vi "Dashboard Main.vi"() -> ()   [LabVIEW 2011]
panel:
  out "Shoot Now!":bool
  out "Shooter Angle":dbl
  out "Potentiometer":cluster{"Pot Raw":dbl, "Pot Angle":dbl}
  out "Locked On":bool
  out "Indexer":T1
  out "Shooter RPM":dbl
  out "Loaded":bool
  in  "Viewer 2":enum32{"Camera Image 2"}(tab)
  in  "Video Enable 2":bool=TRUE
  out "Camera Image 3":T2(plugin-control)
  out "Image Error Message 2":string="Timeout in Camera Communications"
  out "Bridge Balanced":bool
  out "CountDown":dbl format="%#_5g"
  out "Camera":T3
  in  "Viewer":enum32{"Camera Image"}(tab)
  in  "Video Enable":bool=TRUE
  out "Camera Image":T2(plugin-control)
  out "Dashboard Datatype Warning":string="Warning: The Dashboard Datatype used by the robot project and this dashboard do not match.\nSee diagram for more details."
  out "Robot IP Address":string
  out "Image Error Message":string="Timeout in Camera Communications"
  # "Communications"
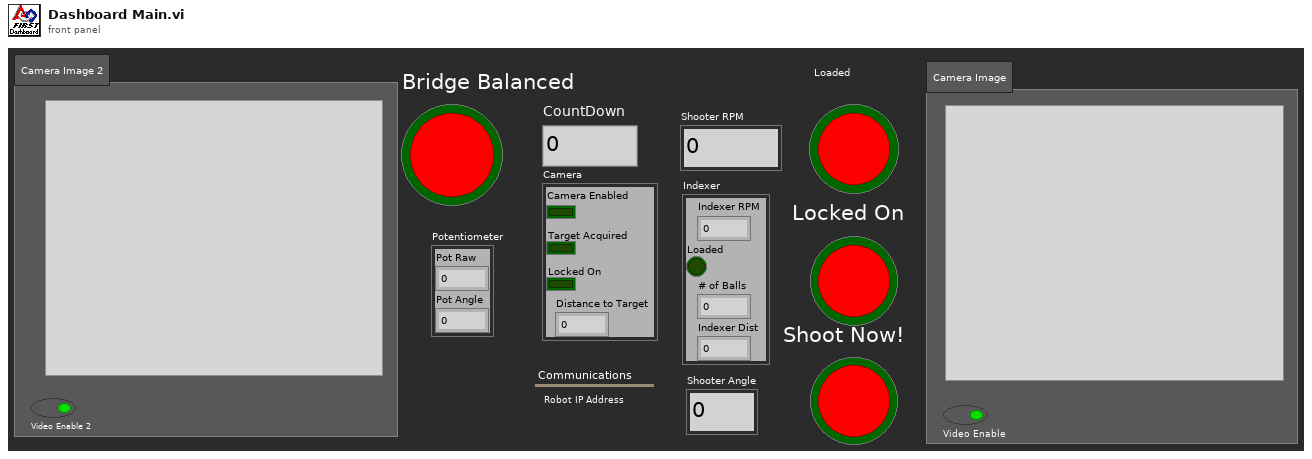
[diagram p1: front panel]
types:
  T1 = cluster{"Indexer RPM":dbl, "Loaded":bool, "# of Balls":dbl, "Indexer Dist":dbl}
  T2 = typedef "IMAQ Image.ctl" = refnum<image>
  T3 = cluster{"Locked On":bool, "Target Acquired":bool, "Camera Enabled":bool, "Distance to Target":dbl}
  T4 = cluster{"Robot Outputs":cluster{"Shooter":cluster{"Shooter RPM":dbl, "Shooter Angle":dbl, "Shooter Power":dbl, "Shooter Enabled":bool}, "Indexer":cluster{"Indexer RPM":dbl, "Loaded":bool, "# of Balls":dbl, "Indexer Dist":dbl}, "Camera":cluster{"Locked On":bool, "Target Acquired":bool, "Camera Enabled":bool, "Distance to Target":dbl}, "Potentiometer":cluster{"Pot Raw":dbl, "Pot Angle":dbl}, "Others":cluster{"CountDown":dbl, "Bridge Balance":bool, "PID Stable":bool}}}
  T5 = typedef "Image Type" = u32
  T6 = typedef "LVRectTypeDef.ctl" = cluster{"left":i16, "top":i16, "right":i16, "bottom":i16}
  T7 = cluster{"Competition mode":bool, "Robot Link":bool, "Autonomous":bool, "Enabled":bool, "E-Stop":bool}
  T8 = cluster{"Shooter":cluster{"Shooter RPM":dbl, "Shooter Angle":dbl, "Shooter Power":dbl, "Shooter Enabled":bool}, "Indexer":cluster{"Indexer RPM":dbl, "Loaded":bool, "# of Balls":dbl, "Indexer Dist":dbl}, "Camera":cluster{"Locked On":bool, "Target Acquired":bool, "Camera Enabled":bool, "Distance to Target":dbl}, "Potentiometer":cluster{"Pot Raw":dbl, "Pot Angle":dbl}, "Others":cluster{"CountDown":dbl, "Bridge Balance":bool, "PID Stable":bool}}
  T9 = cluster{"Shooter RPM":dbl, "Shooter Angle":dbl, "Shooter Power":dbl, "Shooter Enabled":bool}
  T10 = cluster{"CountDown":dbl, "Bridge Balance":bool, "PID Stable":bool}
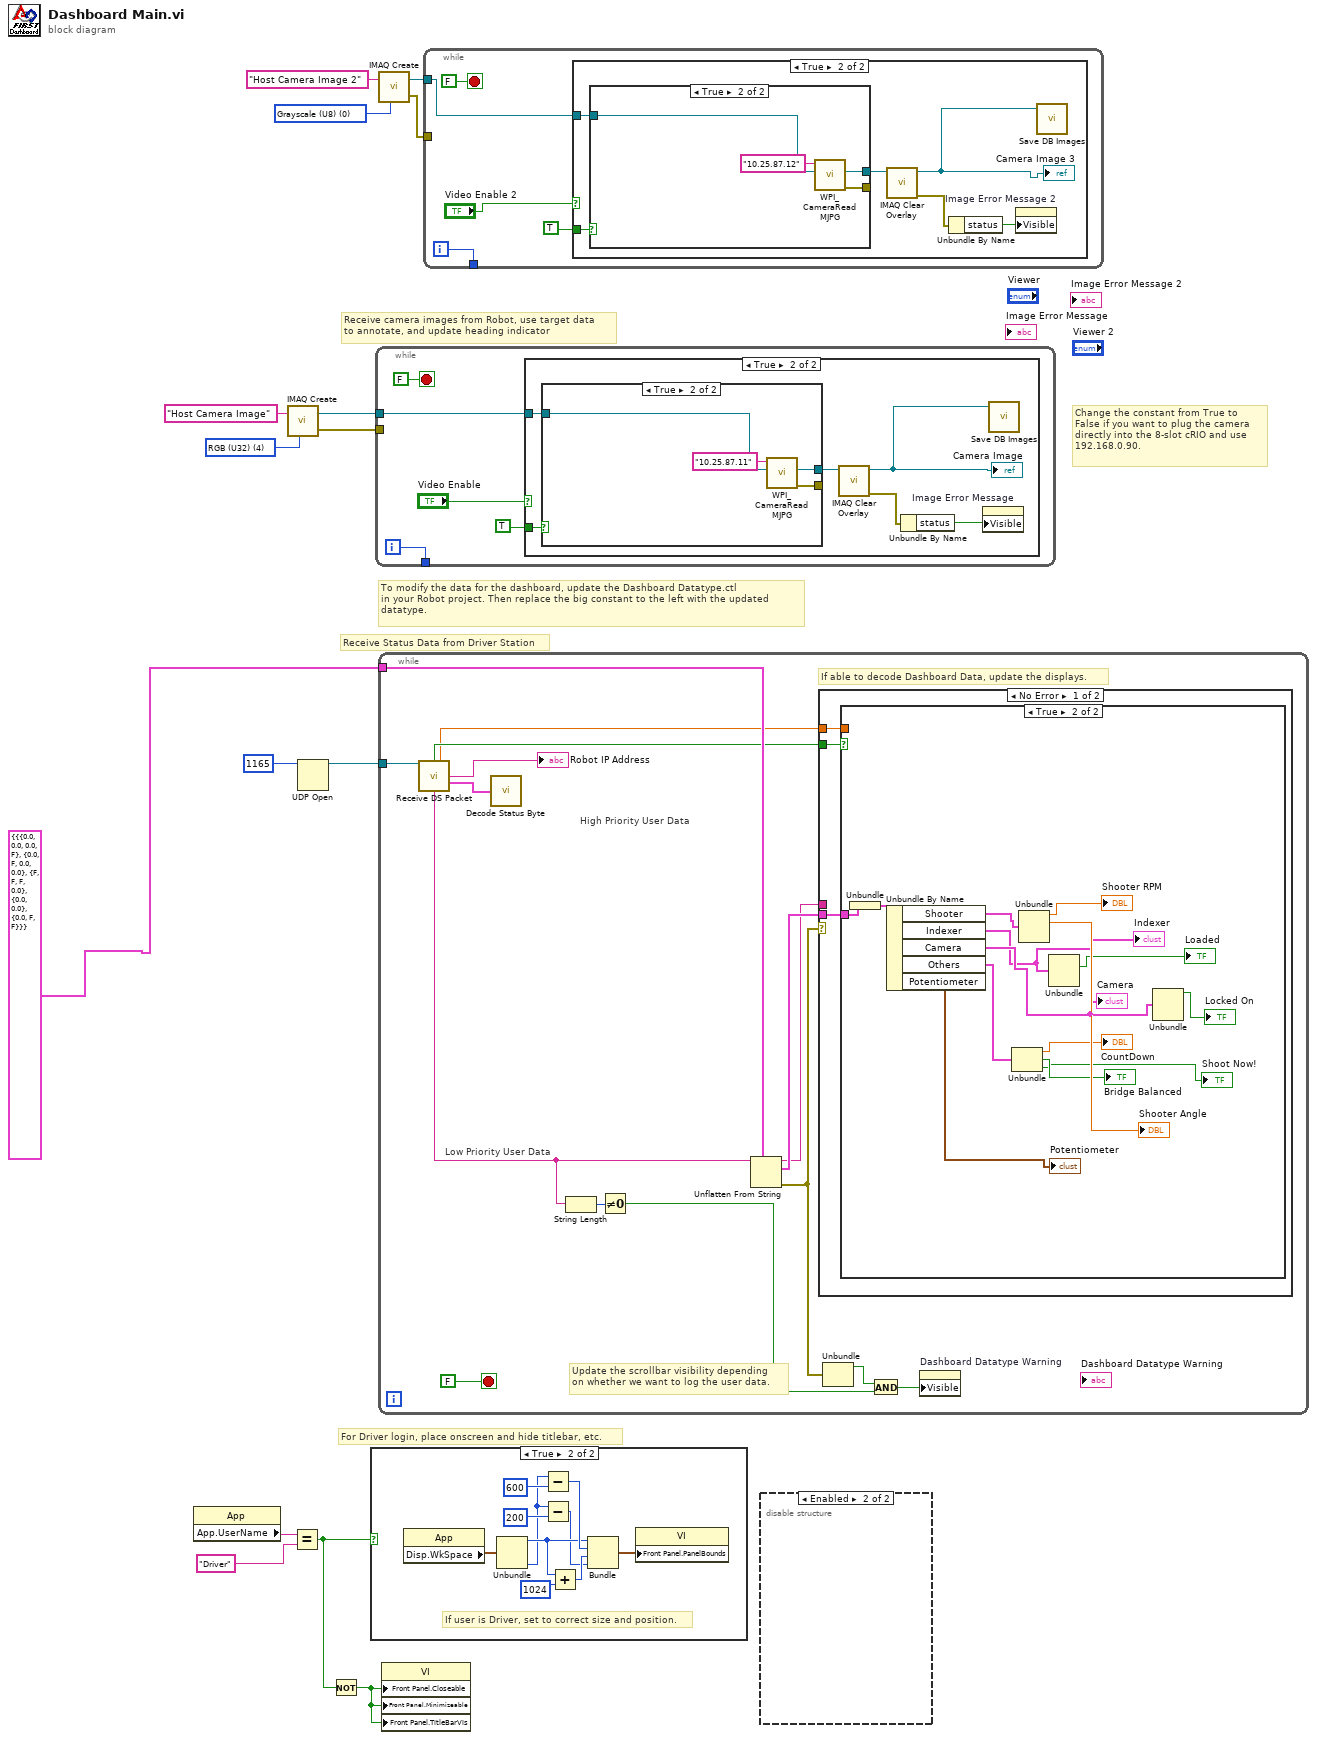
[diagram p0: block diagram]
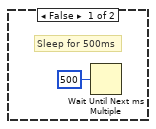
[diagram p2: hidden frame]
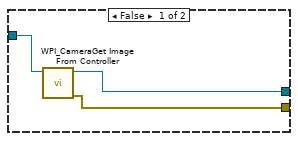
[diagram p3: hidden frame]
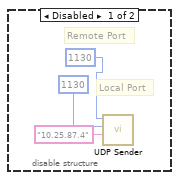
[diagram p4: hidden frame]
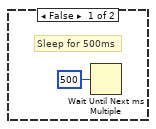
[diagram p8: hidden frame]
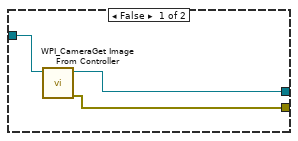
[diagram p9: hidden frame]
diagram:
  w5 = T5 0 items=["Grayscale (U8)", "Grayscale (I16)", "Grayscale (SGL)", "Complex (CSG)", "RGB (U32)", "HSL (U32)", "RGB (U64)"] ("Image Type")
  w13 = T5 4 items=["Grayscale (U8)", "Grayscale (I16)", "Grayscale (SGL)", "Complex (CSG)", "RGB (U32)", "HSL (U32)", "RGB (U64)"] ("Image Type")
  # "Change the constant from True to\nFalse if you want to plug the camera\ndirectly into the 8-slot cRIO and use\n192.168.0.90."
  # "For Driver login, place onscreen and hide titlebar, etc."
  # "To modify the data for the dashboard, update the Dashboard Datatype.ctl\nin your Robot project. Then replace the big constant to the left with the updated\ndatatype."
  # "Receive Status Data from Driver Station"
  # "Receive camera images from Robot, use target data\nto annotate, and update heading indicator"
  n1 = property class="App"() -> ("App.UserName"=w8:string)  [unwired: 2 in, 2 out]
  n2 = call "IMAQ Create"("Image Name"="Host Camera Image", "Image Type"=w13) -> ("New Image"=w11:T2, "error out"=w10:errorcluster)  [unwired: 2 in, 1 out]
  n3 = Equal?(x=w8, y="Driver") -> (x = y?=w7:bool)
  n4 = UDP Open(11:u16 1165 ("port")) -> (port=w14:refnum<k16>)  [unwired: 2 in, 4 out]
  n5 = Not(x=w7) -> (.not. x?=w6:bool)
  n6 = case shown="True" w7 {
    frame False {
    }
    frame True {
      # "If user is Driver, set to correct size and position."
      n7 = property class="App"() -> ("Disp.WkSpace"=w25:T6)  [unwired: 2 in, 2 out]
      n8 = Unbundle(w25) -> ("left"=w20:i16, "bottom"=w16:i16)  [unwired: 2 out]
      n9 = Subtract(x=w16, y=600) -> (x-y=w22:i32)
      n10 = Subtract(x=w16, y=200) -> (x-y=w17:i32)
      n11 = Add(x=w20, y=1024) -> (x+y=w21:i32)
      n12 = Bundle("left"=w20, w22, w21, w17) -> (w24:cluster{"left":i16, i32, i32, i32})  [unwired: 1 out]
      n13 = property class="VI"("Front Panel.PanelBounds"=w24) -> ()  [unwired: 2 in, 2 out]
    }
  }
  n14 = while {
    tunnel: w11 -> [w29]
    tunnel: w10 -> [_]
    tunnel: [w26] -> _
    i -> [w26]
    stop <- FALSE stop-if-true
    n15 = case shown="True" "Video Enable" {
      tunnel: w29 -> [_ w37]
      tunnel: TRUE -> [_ w34]
      frame False {
        # "Sleep for 500ms"
        n16 = Wait Until Next ms Multiple(millisecond multiple=u32 500) -> ()  [unwired: 1 out]
      }
      frame True {
        n17 = case shown="True" w34 {
          tunnel: w37 -> [w40 w44]
          tunnel: [w38 w42] -> _
          tunnel: [w39 w43] -> w35
          frame False {
            n18 = call <vilib>:"WPI_CameraGet Image From Controller.vi"("Image"=w40) -> ("error out"=w38:errorcluster, "Image Out"=w39:T2)  [unwired: 3 in, 6 out]
          }
          frame True {
            n19 = call <vilib>:"WPI_CameraRead MJPG.vi"("Image"=w44, "address"="10.25.87.11") -> ("error out"=w42:errorcluster, "Image Out"=w43:T2)  [unwired: 8 in]
          }
        }
        n20 = call "IMAQ Clear Overlay"("Image"=w35) -> ("error out"=w36:errorcluster, "Image Out"=w32:T2)  [unwired: 2 in, 7 out]
        "Camera Image" <- w32
        n21 = Unbundle By Name(w36) -> ("status"=w33:bool)
        n22 = property on="Image Error Message" class="Str"("Visible"=w33) -> ()  [unwired: 2 in, 2 out]
        n23 = call "Save DB Images.vi"("Image"=w32) -> ()  [unwired: 2 in, 1 out]
      }
    }
  }
  n24 = call "IMAQ Create"("Image Name"="Host Camera Image 2", "Image Type"=w5) -> ("New Image"=w3:T2, "error out"=w2:errorcluster)  [unwired: 2 in, 1 out]
  n25 = while {
    tunnel: w14 -> [w57]
    tunnel: T4 {"Robot Outputs"={"Shooter"={"Shooter RPM"=0.0, "Shooter Angle"=0.0, "Shooter Power"=0.0, "Shooter Enabled"=FALSE}, "Indexer"={"Indexer RPM"=0.0, "Loaded"=FALSE, "# of Balls"=0.0, "Indexer Dist"=0.0}, "Camera"={"Locked On"=FALSE, "Target Acquired"=FALSE, "Camera Enabled"=FALSE, "Distance to Target"=0.0}, "Potentiometer"={"Pot Raw"=0.0, "Pot Angle"=0.0}, "Others"={"CountDown"=0.0, "Bridge Balance"=FALSE, "PID Stable"=FALSE}}} ("Dashboard Data") -> [w56]
    stop <- FALSE stop-if-true
    # "High Priority User Data"
    # "Low Priority User Data"
    # "Update the scrollbar visibility depending\non whether we want to log the user data."
    # "If able to decode Dashboard Data, update the displays."
    n26 = call "Receive DS Packet.vi"("Recv Socket"=w57) -> ("New Dashboard Data"=w53:bool, "Battery"=w45:sgl, "Robot IP Address"=→"Robot IP Address":string, "Status"=w58:T7, "Low Priority User Data"=w46:string)  [unwired: 1 in, 9 out]
    n27 = call "Decode Status Byte.vi"("Status Byte"=w58) -> ()  [unwired: 2 out]
    n28 = String Length(string=w46) -> (length=w48:i32)
    n29 = Not Equal To 0?(x=w48) -> (x != 0?=w51:bool)
    n30 = Unflatten From String(type=w56, binary string=w46) -> (rest of the binary string=w49:string, value=w55:T4, error out=w54:errorcluster)  [unwired: 1 in, 2 out]
    n31 = case shown="No Error" w54 {
      tunnel: w55 -> [w62 _]
      tunnel: w53 -> [w61 _]
      tunnel: w49 -> [_ _]
      tunnel: w45 -> [w60 _]
      frame No Error {
        n32 = case shown="True" w61 {
          tunnel: w62 -> [_ w76]
          tunnel: w60 -> [_ _]
          frame False {
            # "Don't update if the robot hasn't sent new data"
          }
          frame True {
            n33 = Unbundle(w76) -> ("Robot Outputs"=w75:T8)
            n34 = Unbundle By Name(w75) -> ("Shooter"=w74:T9, "Indexer"=w66:T1, "Camera"=w67:T3, "Others"=w71:T10, "Potentiometer"=→"Potentiometer":cluster{"Pot Raw":dbl, "Pot Angle":dbl})
            "Camera" <- w67
            "Indexer" <- w66
            n35 = Unbundle(w71) -> ("CountDown"=→"CountDown":dbl, "Bridge Balance"=→"Bridge Balanced":bool, "PID Stable"=→"Shoot Now!":bool)
            n36 = Unbundle(w74) -> ("Shooter RPM"=→"Shooter RPM":dbl, "Shooter Angle"=→"Shooter Angle":dbl)  [unwired: 2 out]
            n37 = Unbundle(w66) -> ("Loaded"=→"Loaded":bool)  [unwired: 3 out]
            n38 = Unbundle(w67) -> ("Locked On"=→"Locked On":bool)  [unwired: 3 out]
          }
        }
      }
      frame Error {
        # "Your datatypes don't match. The Dashboard Datatype.ctl in your Robot project\nand the big constant to the left of the loop need to match."
      }
    }
    n39 = Unbundle(w54) -> ("status"=w50:bool)  [unwired: 2 out]
    n40 = And(x=w50, y=w51) -> (x .and. y?=w52:bool)
    n41 = property on="Dashboard Datatype Warning" class="Str"("Visible"=w52) -> ()  [unwired: 2 in, 2 out]
  }
  n42 = property class="VI"("Front Panel.Closeable"=w6, "Front Panel.Minimizeable"=w6, "Front Panel.TitleBarVis"=w6) -> ()  [unwired: 2 in, 2 out]
  n43 = while {
    tunnel: [w79] -> _
    tunnel: w3 -> [w78]
    tunnel: w2 -> [_]
    i -> [w79]
    stop <- FALSE stop-if-true
    n44 = case shown="True" "Video Enable 2" {
      tunnel: w78 -> [_ w88]
      tunnel: TRUE -> [_ w85]
      frame False {
        # "Sleep for 500ms"
        n45 = Wait Until Next ms Multiple(millisecond multiple=u32 500) -> ()  [unwired: 1 out]
      }
      frame True {
        n46 = case shown="True" w85 {
          tunnel: w88 -> [w91 w95]
          tunnel: [w89 w93] -> _
          tunnel: [w90 w94] -> w86
          frame False {
            n47 = call <vilib>:"WPI_CameraGet Image From Controller.vi"("Image"=w91) -> ("error out"=w89:errorcluster, "Image Out"=w90:T2)  [unwired: 3 in, 6 out]
          }
          frame True {
            n48 = call <vilib>:"WPI_CameraRead MJPG.vi"("Image"=w95, "address"="10.25.87.12") -> ("error out"=w93:errorcluster, "Image Out"=w94:T2)  [unwired: 8 in]
          }
        }
        n49 = call "IMAQ Clear Overlay"("Image"=w86) -> ("error out"=w87:errorcluster, "Image Out"=w83:T2)  [unwired: 2 in, 7 out]
        "Camera Image 3" <- w83
        n50 = Unbundle By Name(w87) -> ("status"=w84:bool)
        n51 = property on="Image Error Message 2" class="Str"("Visible"=w84) -> ()  [unwired: 2 in, 2 out]
        n52 = call "Save DB Images.vi"("Image"=w83) -> ()  [unwired: 2 in, 1 out]
      }
    }
  }
  n53 = disable-structure shown="Enabled" {
    frame Disabled {
      # "Local Port"
      # "Remote Port"
      n54 = call "UDP Sender.vi"("Remote Host"="10.25.87.4", "Local Port"=u16 1130, "Remote Port"=u16 1130) -> ()  [unwired: 2 in]
    }
    frame Enabled {
    }
  }
